vi "Stop Core.vi"(10 "final error code":i32, 11 "DAQ_Module in":refnum<class "DAQ_Module.lvclass">) -> (3 "DAQ_Module out":refnum<class "DAQ_Module.lvclass">)   [LabVIEW 2025, in "DAQ_Module.lvlib" / "DAQ_Module.lvclass"]
doc: "<p>(<strong>Filename</strong>: <span class=\"dnl\">Actor Framework.lvlib:Actor.lvclass:Stop Core.vi</span>)</p>\n<p>Defines what the actor does before it stops. Use the <strong>final error code</strong> input to determine whether the actor shut down in response to an error.</p>\n<p>By default, this method passes the Stop message along to all <a href=\"nihelplauncher://docs/csh?context=lvcore_lvcomm_af_launch_nested_actor\">auto-stop nested actors</a>. A descendant class may override this method to define additional behavior, such as shutting down any processes the actor initiated in its override of the <a href=\"nihelplauncher://docs/csh?context=lvcore_lvcomm_af_actor_core\">Actor Core</a> method.</p>"
uses:
  DAQ_Module.lvclass
  <vilib>/ActorFramework/Time-Delayed Send Message/Time-Delay Override Options.ctl
  DAQ_Module.lvclass/DAQ_Module.ctl
  Module/Module/Module/Module.lvclass
  <vilib>/ActorFramework/Actor Framework.lvlib
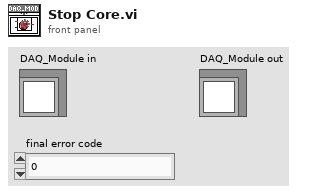
[diagram p1: front panel]
types:
  T1 = typedef "Actor Framework.lvlib/Time-Delay Override Options.ctl" = enum16{"Send next copy now", "Skip next scheduled copy", "Send next copy now and stop all further copies", "Stop all further copies"}
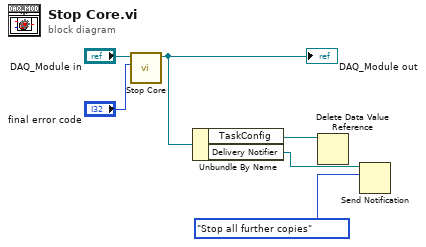
[diagram p0: block diagram]
diagram:
  n1 = call-parent "Stop Core.vi"("final error code"="final error code", "Module in"="DAQ_Module in") -> ("Module out"=w4:refnum<class "DAQ_Module.lvclass">)  [unwired: 9 in]
  "DAQ_Module out" <- w4
  n2 = Unbundle By Name(w4) -> ("TaskConfig"=w3:refnum<data-value>, "Delivery Notifier"=w1:refnum<notifier>)
  n3 = Delete Data Value Reference(data value reference=w3) -> ()  [unwired: 1 in, 2 out]
  n4 = Send Notification(notification=Time-Delay_Override_Options."Stop all further copies", notifier=w1) -> ()  [unwired: 1 in, 2 out]
